vi "S2DS_GR-new.vi"(8 "error in (no error)":errorcluster, 9 "Write command":string, 10 "format string":string, 11 "VISA Refnum in":refnum<visa-resource-name>) -> (0 "error out":errorcluster, 2 "GR 1":dbl, 3 "VISA Refnum out":refnum<visa-resource-name>)   [LabVIEW 2025]
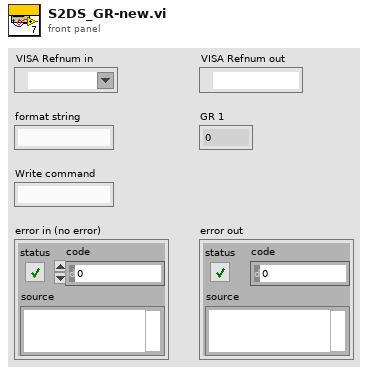
[diagram p1: front panel]
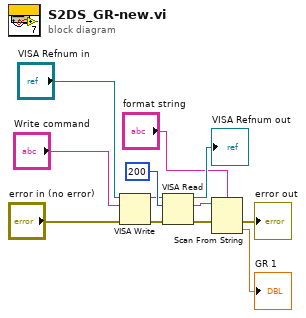
[diagram p0: block diagram]
diagram:
  n1 = VISA Write(VISA resource name="VISA Refnum in", write buffer="Write command", error in (no error)="error in (no error)") -> (VISA resource name out=w3:refnum<visa-resource-name>, error out=w2:errorcluster)  [unwired: 1 out]
  n2 = VISA Read(VISA resource name=w3, byte count=u32 200, error in (no error)=w2) -> (VISA resource name out=→"VISA Refnum out":refnum<visa-resource-name>, read buffer=w5:string, error out=w4:errorcluster)  [unwired: 1 out]
  n3 = Scan From String(format string="format string", input string=w5, error in=w4) -> (error out=→"error out":errorcluster, output 1=→"GR 1":dbl)  [unwired: 2 in, 2 out]
